vi "sub-obtain service info.vi"(7 "Service Name":string, 8 "error in (no error)":errorcluster, 11 "service list":T2(array[cluster])) -> (0 "error out":errorcluster, 2 "Service Info":T1)   [LabVIEW 2016]
doc: "Find the communication parameters for certain service name"
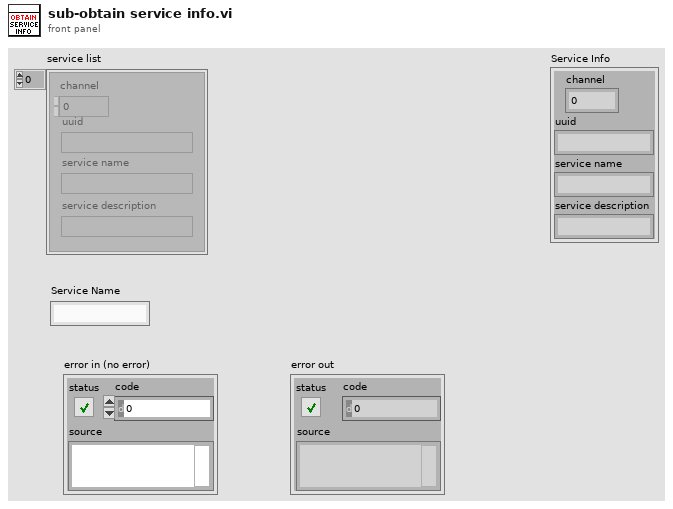
[diagram p1: front panel]
types:
  T1 = cluster{"channel":u16, "uuid":string, "service name":string, "service description":string}
  T2 = cluster{"channel":u16, "uuid":string, "service name":string, "service description":string}[]
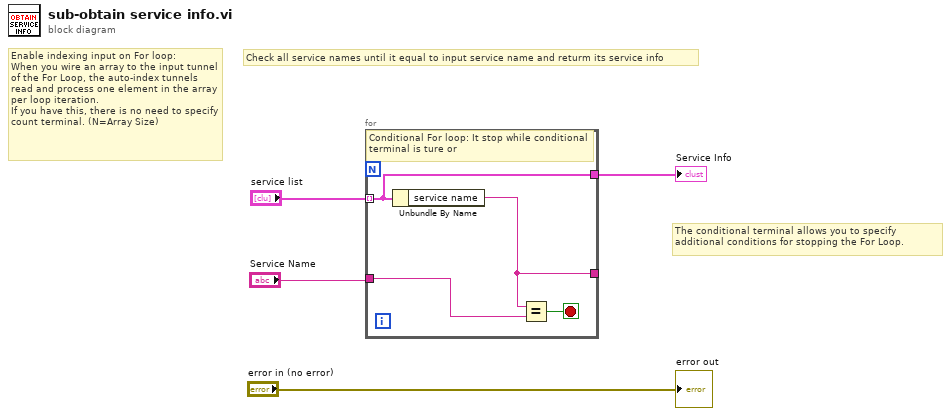
[diagram p0: block diagram]
diagram:
  # "The conditional terminal allows you to specify additional conditions for stopping the For Loop."
  # "Enable indexing input on For loop:\nWhen you wire an array to the input tunnel of the For Loop, the auto-index tunnels read and process one element in the array per loop iteration.\nIf you have this, there is no need to specify count terminal. (N=Array Size)"
  # "Check all service names until it equal to input service name and returm its service info"
  n1 = for {
    tunnel: "service list" -> [w5] mode=indexing
    tunnel: "Service Name" -> [w8]
    tunnel: [w6] -> _
    tunnel: [w5] -> w2
    stop <- w7 stop-if-true
    # "Conditional For loop: It stop while conditional terminal is ture or"
    n2 = Unbundle By Name(w5) -> ("service name"=w6:string)
    n3 = Equal?(x=w6, y=w8) -> (x = y?=w7:bool)
  }
  "Service Info" <- w2
  "error out" <- "error in (no error)"
